vi "RetractCanBurgler.vi"(9 "dt":i32, 10 "SensorInputData":T2, 11 "HMI to Control":T1) -> (2 "SensorInputDataOut":T2, 3 "HMI to ControlOut":T1, 4 "Done":bool=TRUE)   [LabVIEW 2015]
uses:
  Typedefs/SensorInputData.ctl
  Typedefs/HMI_to_Control.ctl
panel:
  in  "arguments":string[](array[string])
  in  "Reinit":bool
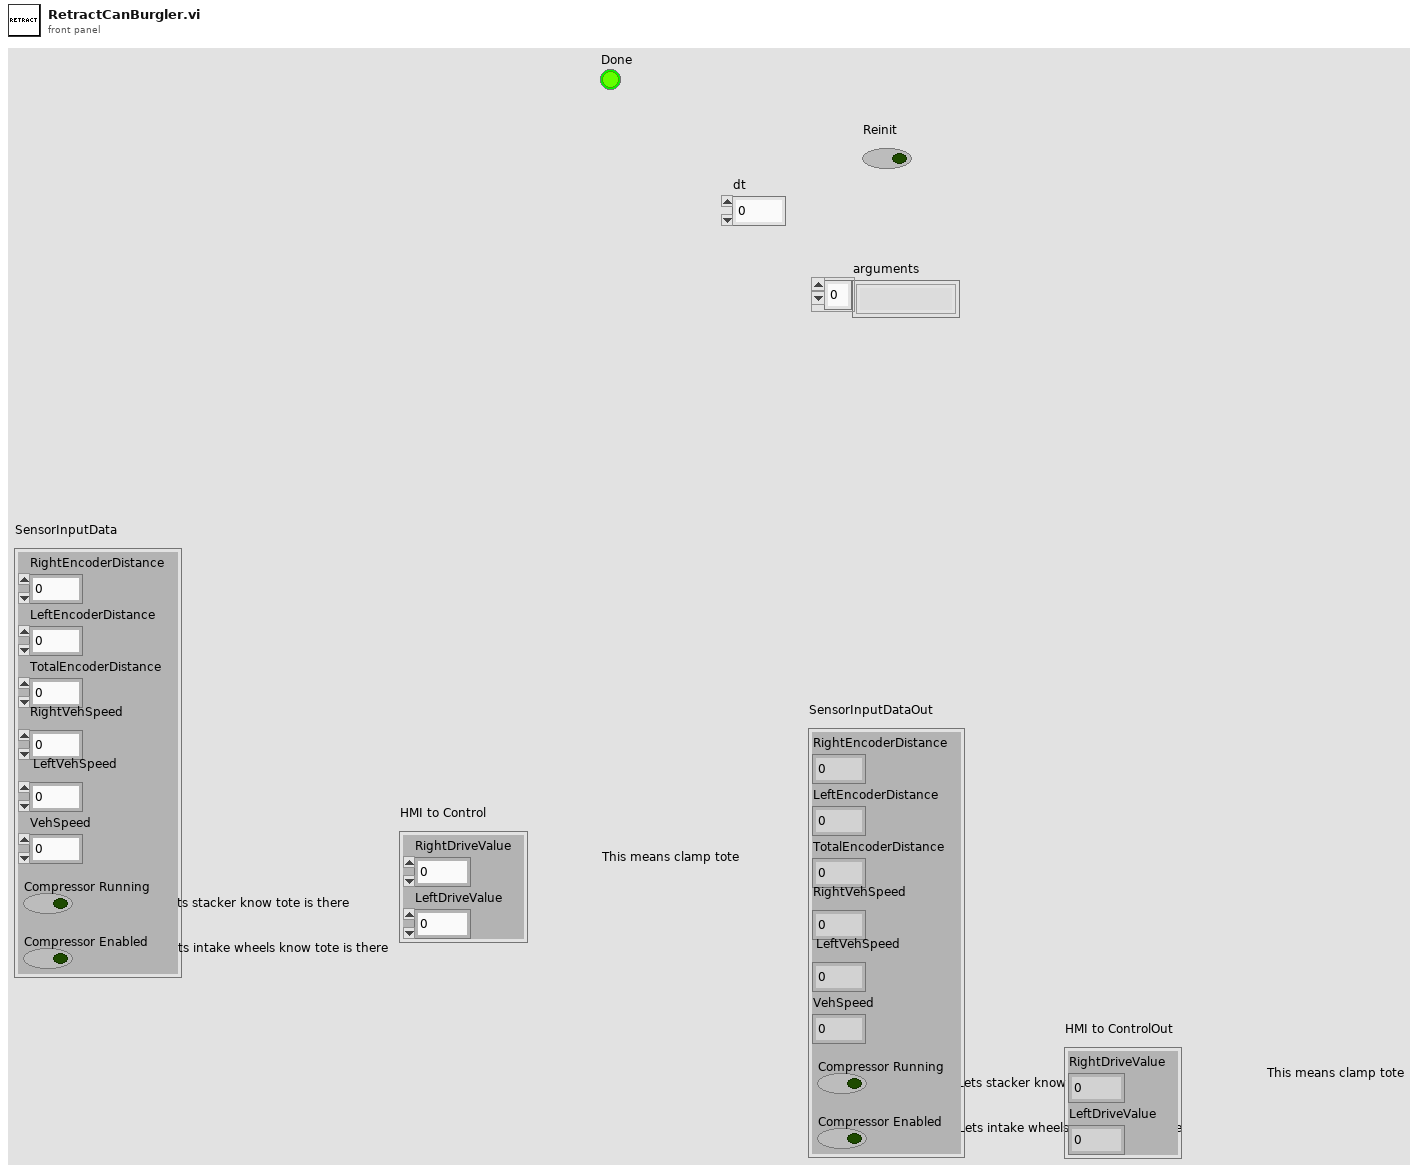
[diagram p1: front panel]
types:
  T1 = typedef "HMI_to_Control.ctl" = cluster{"RightDriveValue":dbl, "LeftDriveValue":dbl}
  T2 = typedef "SensorInputData.ctl" = cluster{"RightEncoderDistance":dbl, "LeftEncoderDistance":dbl, "TotalEncoderDistance":dbl, "RightVehSpeed":dbl, "LeftVehSpeed":dbl, "VehSpeed":dbl, "Compressor Running":bool, "Compressor Enabled":bool}
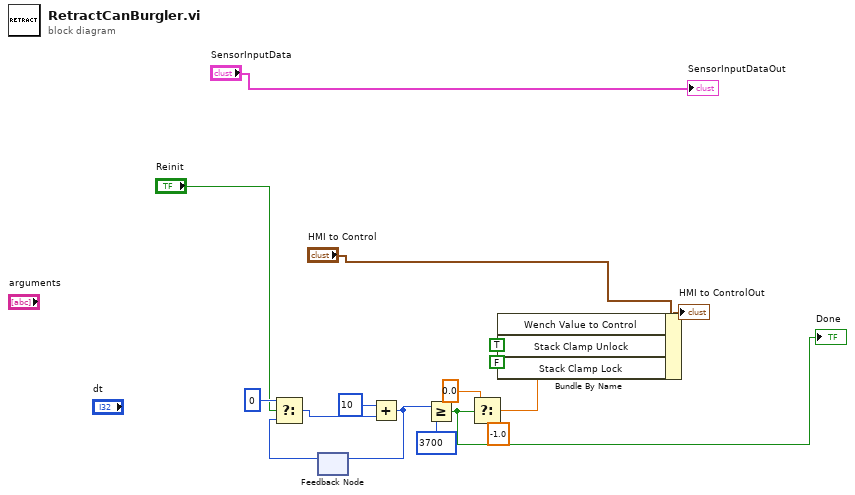
[diagram p0: block diagram]
diagram:
  n1 = feedback #1() -> (w10:i32)  [unwired: 1 in]
  n2 = Select(t=0, s="Reinit", f=w10) -> (s? t:f=w13:i32)
  n3 = Add(x=10, y=w13) -> (x+y=w9:i32)
  n4 = feedback-in #1(w9) -> ()
  n5 = Greater Or Equal?(x=w9, y=3700) -> (x >= y?=w2:bool)
  "Done" <- w2
  n6 = Select(t=0.0, s=w2, f=-1.0) -> (s? t:f=w6:dbl)
  n7 = Bundle By Name(cluster="HMI to Control", "Wench Value to Control"=w6, "Stack Clamp Unlock"=TRUE, "Stack Clamp Lock"=FALSE) -> (→"HMI to ControlOut":T1)
  "SensorInputDataOut" <- "SensorInputData"
